vi "Serial Write and Read Mark-10 Example.vi"(0 "VISA resource name":refnum<visa-resource-name>="COM1", 1 "Baud Rate":u32=115200, 2 "Data Bits":u16=8 min=5 max=8 step=1, 3 "Parity":u16(ring) items=["None", "Odd", "Even", "Mark", "Space"], 4 "Stop Bits":u16(ring)=10 items=["1.0"=10, "1.5"=15, "2.0"=20], 5 "Write & Read":bool=TRUE, 7 "Flow Control":u16(ring) items=["None"=0, "XON/XOFF"=1, "RTS/CTS"=2, "DTR/DSR"=4], 8 "String to Write":string="?\r") -> (9 "Read String":string, 10 "Bytes Read":u32)   [LabVIEW 2016]
doc: "The Basic Serial Read and Write example performs a Serial Port Read, a Serial Port Write, or a combination of these actions. The user selects the actions (read or write) on the front panel. If both are selected, the VI will write the data first, read data, and then close the VISA session that is opened to the port. This VI will wait until the specified number of bytes is received at the port. Only the number of bytes specified will be read.\n\nINSTRUCTIONS:\n1) Select the serial resource and configuration parameters (baud rate, data bits, parity, stop bits, flow control).\n2) Select the operations to be performed. \n3) Connect the serial port to your device. If no device is available, perform a loopback test by doing one of the following. Short pins 2 and 3 on a RS-232 cable or short pin 4 to pin 8 and pin 5 to pin 9 on a RS-485/422 cable. \n4) Run the VI to see the data read. (The \"read string\" will match the \"string to write\" if a loopback test was performed.)\n\nNote: The parameters set for the serial port must match the parameters of the connected instrument or device. In this example, the bytes to read parameter specifies the number of bytes that the serial port reads. If there were more bytes at the port than the number specified in bytes to read, those bytes would not be read. Also, if you specify to read more bytes than the number of bytes actually read, you might receive a timeout error message.\n\nOn the block diagram, the Configure Serial Port VI sets the configuration parameters. The front panel displays the controls used to configure the basic parameters, such as baud rate, data bits, and parity. Constants configure the other parameters the user probably does not need set. After the VISA Configure Serial Port VI opens the VISA session and configures the port, the VI passes the VISA resource name to other VIs that perform operations on that VISA resource. The VISA Write function sends a command to the serial device and the VISA Read function returns data based on the command. The VISA Close function then closes the reference to the serial device. It is important to close the reference; otherwise communication through with that port through protocols other than VISA might not be possible."
uses:
  <vilib>/Instr/_visa.llb/VISA Configure Serial Port (Instr).vi
panel:
  in  "Max Speed":bool
  in  "Apply":bool
  out "Load":cluster{"Y":dbl[], dbl[]}(graph)
  out "Current Reading":string
  out "Iterations / Sec.":dbl
  out "Elapsed Time (sec)":dbl
  out "Iterations":i32
  in  "stop":bool
  in  "Delay Before Read (mS)":u32=50
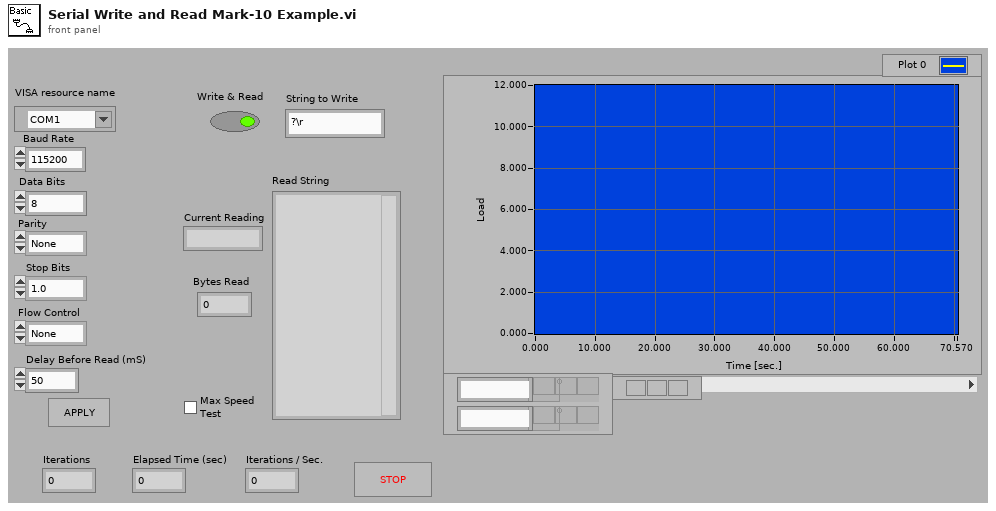
[diagram p1: front panel]
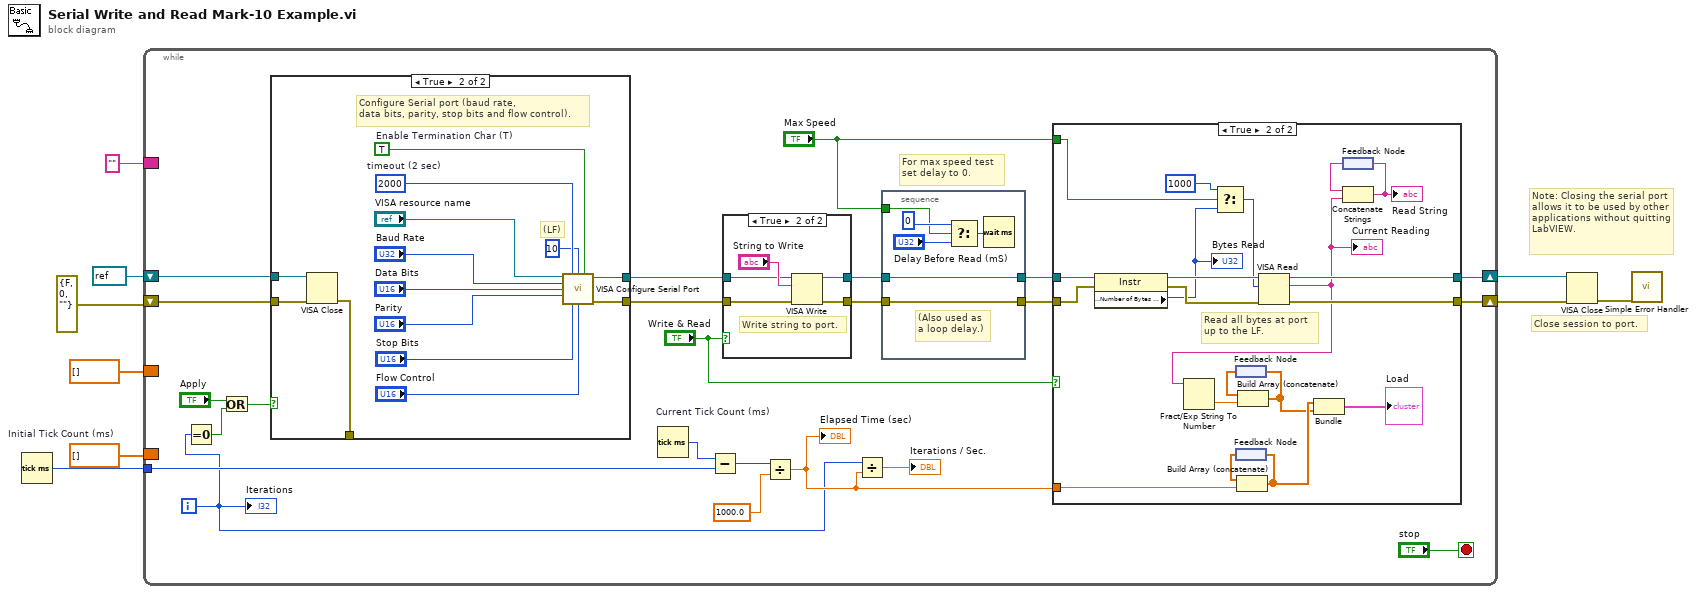
[diagram p0: block diagram]
diagram:
  # "Note: Closing the serial port allows it to be used by other applications without quitting LabVIEW."
  # "Close session to port."
  n1 = Tick Count (ms) "Initial Tick Count (ms)"() -> (millisecond timer value=w6:u32)
  n2 = while {
    tunnel: w6 -> [w22]
    border: "" -> [_]
    border: dbl[] [] -> [_]
    border: dbl[] [] -> [_]
    shift-right: [w27] -> w8
    shift-left: refnum<visa-resource-name> refnum ("VISA resource name out") -> [w16]
    shift-right: [w28] -> w7
    shift-left: errorcluster {"status"=FALSE, "code"=0, "source"=""} ("error out") -> [w15]
    i -> [w12]
    stop <- "stop" stop-if-true
    # "For max speed test \nset delay to 0."
    n3 = Equal To 0?(x=w12) -> (x = 0?=w13:bool)
    n4 = Or(x="Apply", y=w13) -> (x .or. y?=w14:bool)
    n5 = case shown="True" w14 {
      tunnel: [w56 w61] -> w19
      tunnel: [w55 w60] -> w18
      tunnel: w16 -> [w56 w59]
      tunnel: w15 -> [w55 w58]
      tunnel: [_ w57] -> _
      frame False {
      }
      frame True {
        w66 = TRUE  # Enable Termination Char (T)
        w67 = u32 2000  # timeout (2 sec)
        # "(LF)"
        # "Configure Serial port (baud rate,\ndata bits, parity, stop bits and flow control)."
        n6 = VISA Close(VISA resource name=w59, error in (no error)=w58) -> (error out=w57:errorcluster)
        n7 = call-poly "VISA Configure Serial Port"("VISA resource name"="VISA resource name", "timeout (10sec)"=w67, "termination char\n(0xA = '\\n' = LF)"=u8 10 ("termination char\n(0xA = '\\n' = LF)"), "Enable Termination\nChar (T)"=w66, "baud rate (9600)"="Baud Rate", "data bits (8)"="Data Bits", "parity (0:none)"="Parity", "stop bits (10: 1 bit)"="Stop Bits", "flow control (0:none)"="Flow Control") -> ("VISA resource name out"=w61:refnum<visa-resource-name>, "error out"=w60:errorcluster)  [unwired: 5 in]
      }
    }
    n8 = Tick Count (ms) "Current Tick Count (ms)"() -> (millisecond timer value=w25:u32)
    n9 = Subtract(x=w25, y=w22) -> (x-y=w24:u32)
    n10 = case shown="True" "Write & Read" {
      tunnel: [w78 w83] -> w32
      tunnel: w19 -> [w77 w81]
      tunnel: w18 -> [w78 w80]
      tunnel: [w77 w79] -> w30
      frame False {
      }
      frame True {
        # "Write string to port."
        n11 = VISA Write(VISA resource name=w81, write buffer="String to Write", error in (no error)=w80) -> (VISA resource name out=w79:refnum<visa-resource-name>, error out=w83:errorcluster)  [unwired: 1 out]
      }
    }
    n12 = Divide(x=w24, y=1000.0) -> (x/y=w20:dbl)
    "Elapsed Time (sec)" <- w20
    n13 = Divide(x=w12, y=w20) -> (x/y=→"Iterations / Sec.":dbl)
    n14 = stacked-sequence {
      tunnel: w32 -> [w76]
      tunnel: [w76] -> w31
      tunnel: w30 -> [w75]
      tunnel: [w75] -> w29
      tunnel: "Max Speed" -> [w71]
      frame #0 {
        # "(Also used as\na loop delay.)"
        n15 = Select(t=u32 0, s=w71, f="Delay Before Read (mS)") -> (s? t:f=w74:u32)
        n16 = Wait (ms)(milliseconds to wait=w74) -> ()  [unwired: 1 out]
      }
    }
    n17 = case shown="True" "Write & Read" {
      tunnel: w31 -> [w33 w54]
      tunnel: w29 -> [w34 w53]
      tunnel: [w33 w52] -> w28
      tunnel: [w34 w51] -> w27
      tunnel: w20 -> [_ w44]
      tunnel: "Max Speed" -> [_ w37]
      frame False {
      }
      frame True {
        # "Read all bytes at port\nup to the LF."
        n18 = property class="Instr"(reference=w53, error in=w54) -> (reference out=w50:refnum<visa-resource-name>, error out=w49:errorcluster, "Serial Settings:Number of Bytes at Serial Port"=w36:u32)
        "Bytes Read" <- w36
        n19 = Select(t=u32 1000 ("byte count"), s=w37, f=w36) -> (s? t:f=w35:u32)
        n20 = feedback #1() -> (w39:dbl[])
        n21 = feedback #2() -> (w41:dbl[])
        n22 = Build Array (concatenate)(w41, w44) -> (w42:dbl[])
        n23 = feedback-in #2(w42) -> ()
        n24 = VISA Read(VISA resource name=w50, byte count=w35, error in (no error)=w49) -> (VISA resource name out=w51:refnum<visa-resource-name>, read buffer=w46:string, error out=w52:errorcluster)  [unwired: 1 out]
        "Current Reading" <- w46
        n25 = Fract/Exp String To Number(string=w46) -> (number=w45:dbl)  [unwired: 3 in, 1 out]
        n26 = Build Array (concatenate)(w39, w45) -> (w40:dbl[])
        n27 = feedback-in #1(w40) -> ()
        n28 = Bundle(w42, w40) -> (→"Load":cluster{dbl[], dbl[]})  [unwired: 1 in]
        n29 = feedback #3() -> (w47:string)
        n30 = Concatenate Strings(w47, w46) -> (w48:string)
        "Read String" <- w48
        n31 = feedback-in #3(w48) -> ()
      }
    }
    "Iterations" <- w12
  }
  n32 = VISA Close(VISA resource name=w8, error in (no error)=w7) -> (error out=w9:errorcluster)
  n33 = call <vilib>:"Simple Error Handler.vi"("error in (no error)"=w9) -> ()  [unwired: 4 in, 5 out]
